vi "Configure DUT Sensor Type.vi"(8 "error in (no error)":errorcluster, 9 "DUT Sensor Type (0)":i16 min=0 max=2 step=1, 11 "VISA resource name":refnum<visa-resource-name>) -> (0 "error out":errorcluster, 3 "VISA resource name out":refnum<visa-resource-name>)   [LabVIEW 2010, in "Temptronic TP04300.lvlib"]
doc: "This control configures DUT sensor type for TP04300 instrument.\n\n<b>DUT Sensor Type</b> as follows:\n 0 - no DUT sensor selected\n 1 - type T thermocouple\n 2 - type K thermocouple\n 3 - RTD\n 4 - diode\n\nDefault Value: 0\nValid Range: 0 - 4"
uses:
  Temptronic TP04300.lvlib
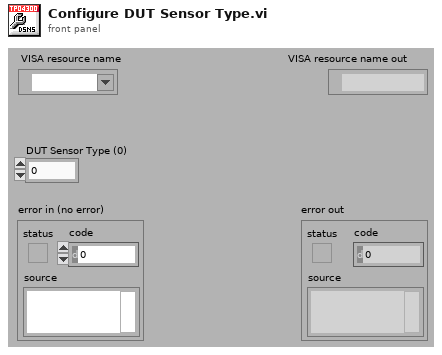
[diagram p1: front panel]
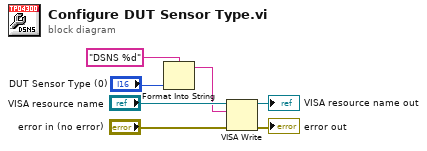
[diagram p0: block diagram]
diagram:
  n1 = Format Into String(format string="DSNS %d" ("multi-line string"), "DUT Sensor Type (0)") -> (resulting string=w3:string)  [unwired: 2 in, 1 out]
  n2 = VISA Write(VISA resource name="VISA resource name", write buffer=w3, error in (no error)="error in (no error)") -> (VISA resource name out=→"VISA resource name out":refnum<visa-resource-name>, error out=→"error out":errorcluster)  [unwired: 1 out]
